vi "Operator Input with validation.vi"(8 "error in (no error)":errorcluster, 10 "Validation string":string, 11 "Message":string) -> (0 "error out":errorcluster, 2 "Stop button hit":bool, 3 "Response":string)   [LabVIEW 2013]
panel:
  out "Data type string":string
  in  "stop":bool
  in  "Response1":string
  # "Operator Message"
  # "Data format"
  # "Scan or Enter Response"
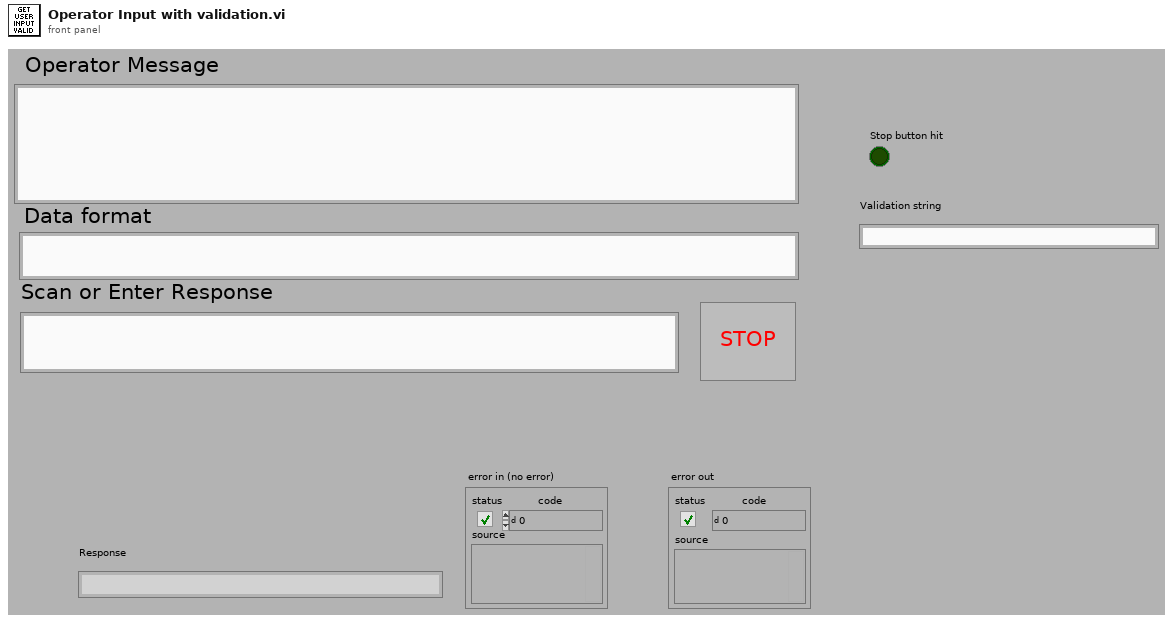
[diagram p1: front panel]
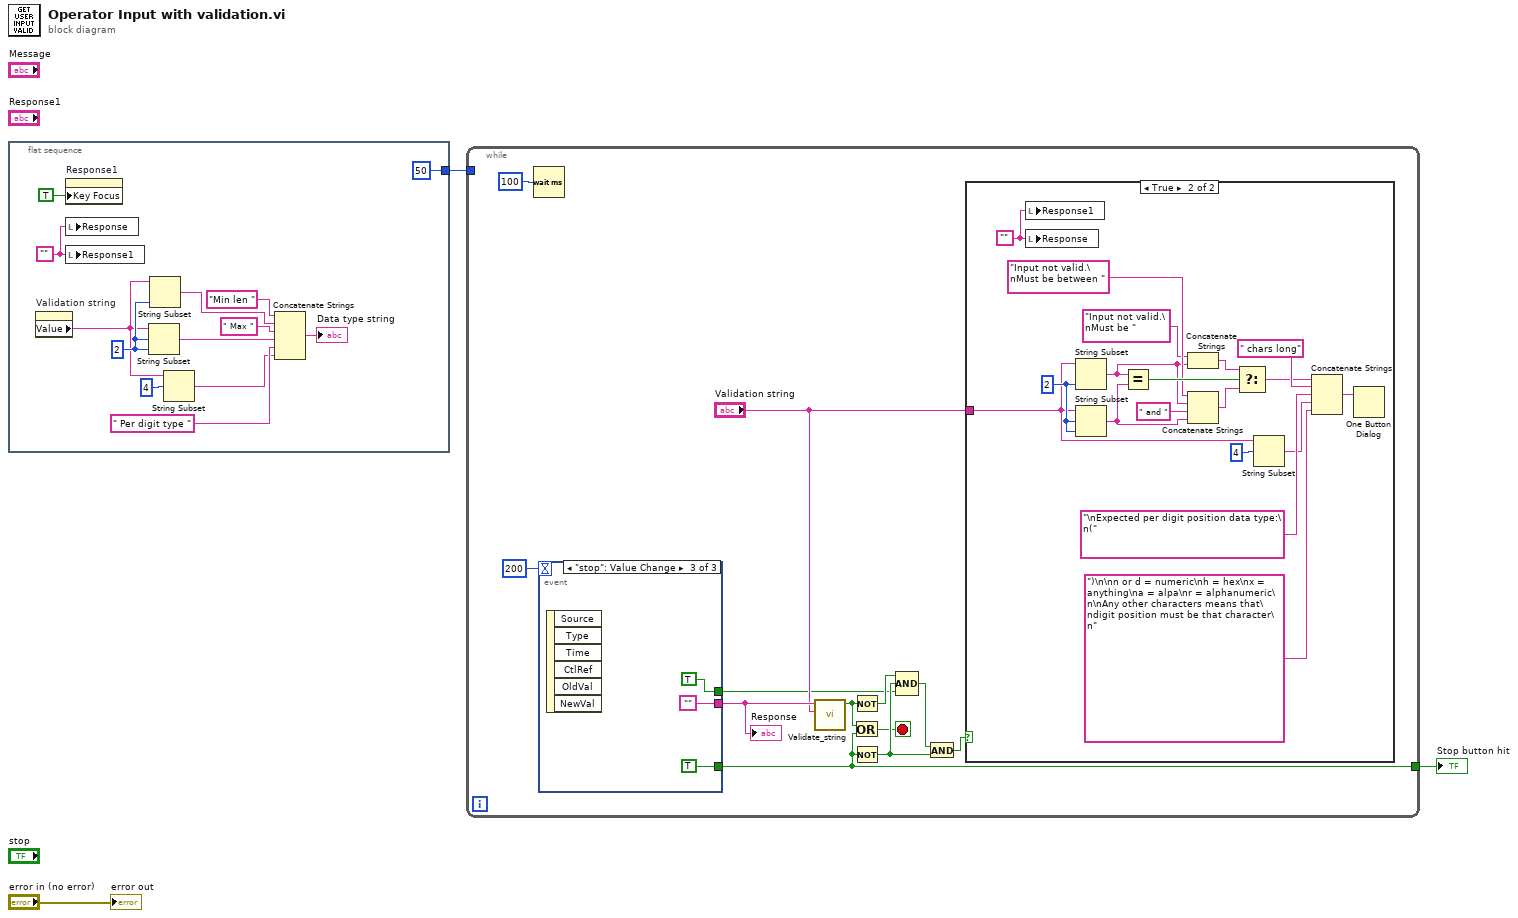
[diagram p0: block diagram]
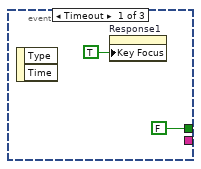
[diagram p3: hidden frame]
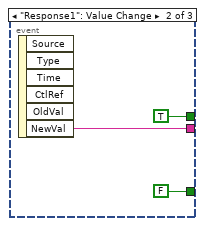
[diagram p4: hidden frame]
diagram:
  n1 = flat-sequence {
    tunnel: [u32 50 ("milliseconds to wait")] -> w3
    frame #0 {
      w10 = 2 ("length (rest)")
      w14 = ""
      n2 = property on="Validation string" class="Str"() -> ("Value"=w7:string)  [unwired: 2 in, 2 out]
      n3 = property on="Response1" class="Str"("Key Focus"=TRUE) -> ()  [unwired: 2 in, 2 out]
      n4 = local write "Response"(w14) -> ()
      n5 = local write "Response1"(w14) -> ()
      n6 = String Subset(string=w7, offset (0)=w10, length (rest)=w10) -> (substring=w9:string)
      n7 = String Subset(string=w7, length (rest)=w10) -> (substring=w11:string)  [unwired: 1 in]
      n8 = String Subset(string=w7, offset (0)=4) -> (substring=w5:string)  [unwired: 1 in]
      n9 = Concatenate Strings("Min len " ("string"), w11, " Max " ("string"), w9, " Per digit type " ("string"), w5) -> (→"Data type string":string)
    }
  }
  n10 = while {
    tunnel: w3 -> [_]
    tunnel: [w18] -> w1
    stop <- w17 stop-if-true
    n11 = Wait (ms)(milliseconds to wait=u32 100) -> ()  [unwired: 1 out]
    n12 = event shown="[2] \"stop\": Value Change" {
      selector: _ -> [_ _ _]
      dyn-events: _ -> [_ _ _]
      timeout: 200 -> [_ _ _]
      tunnel: [FALSE ("Key Focus") TRUE TRUE] -> w22
      tunnel: [_ w50 ""] -> w28
      tunnel: [_ FALSE TRUE] -> w18
      event Timeout {
        n13 = event-data() -> ()  [unwired: 1 in, 2 out]
        n14 = property on="Response1" class="Str"("Key Focus"=TRUE) -> ()  [unwired: 2 in, 2 out]
      }
      event "Response1": Value Change {
        n15 = event-data() -> ("NewVal"=w50:string)  [unwired: 1 in, 5 out]
      }
      event "stop": Value Change {
        n16 = event-data() -> ()  [unwired: 1 in, 6 out]
      }
    }
    "Response" <- w28
    n17 = call "Validate_string.vi"("String data format"="Validation string", "String"=w28) -> ("String Valid"=w19:bool)  [unwired: 8 in, 1 out]
    n18 = Not(x=w19) -> (.not. x?=w24:bool)
    n19 = Or(x=w19, y=w18) -> (x .or. y?=w17:bool)
    n20 = Not(x=w18) -> (.not. x?=w23:bool)
    n21 = Compound Arithmetic op=AND(w24, w23, w22) -> (w21:bool)
    n22 = And(x=w21, y=w23) -> (x .and. y?=w26:bool)
    n23 = case shown="True" w26 {
      tunnel: "Validation string" -> [_ w43]
      frame False {
      }
      frame True {
        w36 = ""
        w46 = 2 ("length (rest)")
        n24 = local write "Response1"(w36) -> ()
        n25 = local write "Response"(w36) -> ()
        n26 = String Subset(string=w43, length (rest)=w46) -> (substring=w34:string)  [unwired: 1 in]
        n27 = String Subset(string=w43, offset (0)=w46, length (rest)=w46) -> (substring=w32:string)
        n28 = Equal?(x=w34, y=w32) -> (x = y?=w38:bool)
        n29 = Concatenate Strings("Input not valid.\nMust be " ("string"), w34) -> (w30:string)
        n30 = Concatenate Strings("Input not valid.\nMust be between " ("string"), w34, " and " ("string"), w32) -> (w31:string)
        n31 = Select(t=w30, s=w38, f=w31) -> (s? t:f=w29:string)
        n32 = String Subset(string=w43, offset (0)=4) -> (substring=w41:string)  [unwired: 1 in]
        n33 = Concatenate Strings(w29, " chars long" ("string"), "\nExpected per digit position data type:\n(" ("string"), w41, ")\n\nn or d = numeric\nh = hex\nx = anything\na = alpa\nr = alphanumeric\n\nAny other characters means that\ndigit position must be that character\n" ("string")) -> (w40:string)
        n34 = One Button Dialog(message=w40) -> ()  [unwired: 1 in, 1 out]
      }
    }
  }
  "Stop button hit" <- w1
  "error out" <- "error in (no error)"
